vi "VCS Get Motor Parameter.vi"(8 "error in (no error)":errorcluster, 11 "axis in":cluster{"keyHandle":u32, "nodeId":u16}={"keyHandle"=0, "nodeId"=1}) -> (0 "error out":errorcluster, 2 "motor Data":T1={"motor Type"=1, "continuousCurrent"=1000, "peakCurrent"=1000, "polePair"=1, "thermalTimeConstant"=40} {"motor Type" items=["Phase modulated DC motor "=1, "Sinusoidal PM BL motor"=10, "Trapezoidal PM BL motor"=11]}, 3 "axis out":cluster{"keyHandle":u32, "nodeId":u16}={"keyHandle"=0, "nodeId"=1})   [LabVIEW 2017, in "maxonEPOS.lvlib"]
doc: "<B>VCS Get Motor Parameter</B> reads all motor parameters."
uses:
  Examples/maxonEPOS.lvlib
  SSI_Tool/InstrumentsInterfaces/Motordriver/maxon EPOS/Resources/EposCmd.dll
  SSI_Tool/InstrumentsInterfaces/Motordriver/maxon EPOS/Resources/EposCmd64.dll
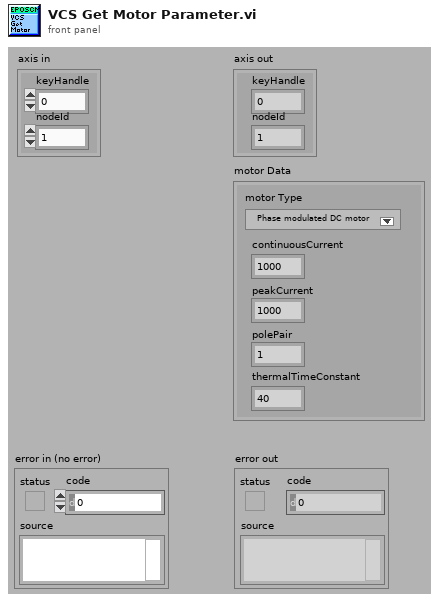
[diagram p1: front panel]
types:
  T1 = cluster{"motor Type":u16, "continuousCurrent":u16, "peakCurrent":u16, "polePair":u8, "thermalTimeConstant":u16}
  T2 = cluster{"pMotorType":u16, "pContinuousCurrent":u16, "pPeakCurrent":u16, "pPolePair":u8, "pThermalTimeConstant":u16}
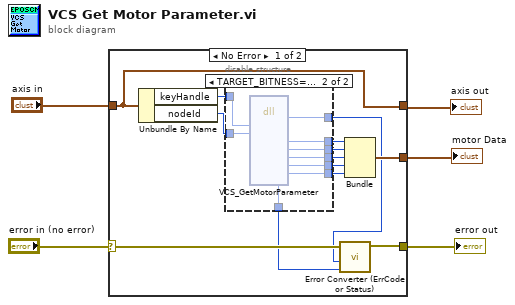
[diagram p0: block diagram]
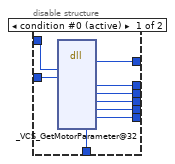
[diagram p2: hidden frame]
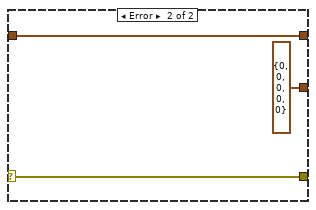
[diagram p3: hidden frame]
diagram:
  n1 = case shown="No Error" "error in (no error)" {
    selector: "error in (no error)" -> [w18 w39]
    tunnel: [w17 w39] -> w4
    tunnel: "axis in" -> [w12 w37]
    tunnel: [w13 T2 {"pMotorType"=0, "pContinuousCurrent"=0, "pPeakCurrent"=0, "pPolePair"=0, "pThermalTimeConstant"=0}] -> w1
    tunnel: [w12 w37] -> w2
    frame No Error {
      n2 = Unbundle By Name(w12) -> ("keyHandle"=w15:u32, "nodeId"=w14:u16)
      n3 = disable-structure shown="TARGET_BITNESS==64" {
        disable-tunnel: [w27 w36] -> w16
        disable-tunnel: w15 -> [w26 w35]
        disable-tunnel: w14 -> [w25 w34]
        disable-tunnel: [w24 w33] -> w11
        disable-tunnel: [w23 w32] -> w10
        disable-tunnel: [w22 w31] -> w9
        disable-tunnel: [w21 w30] -> w8
        disable-tunnel: [w20 w29] -> w7
        disable-tunnel: [w19 w28] -> w6
        frame condition #0 (active) {
          n4 = dll-call lib="C:/workspace/project/scancon/sw/SSI_Tool/InstrumentsInterfaces/Motordriver/maxon EPOS/Resources/EposCmd.*" fn="_VCS_GetMotorParameter@32"("KeyHandle"=w26, "NodeId"=w25) -> (w19:i32, "pMotorType"=w24:u16, "pContinuousCurrent"=w23:u16, "pPeakCurrent"=w22:u16, "pPolePair"=w21:u8, "pThermalTimeConstant"=w20:u16, "pErrorCode"=w27:u32)  [unwired: 11 in, 2 out]
        }
        frame condition #1 {
          n5 = dll-call lib="C:/setup/Resources/EposCmd64.*" fn="VCS_GetMotorParameter" ("EposCmd.dll:_VCS_GetMotorParameter@32")("KeyHandle"=w35, "NodeId"=w34) -> ("Rückgabetyp"=w28:i32, "pMotorType"=w33:u16, "pContinuousCurrent"=w32:u16, "pPeakCurrent"=w31:u16, "pPolePair"=w30:u8, "pThermalTimeConstant"=w29:u16, "pErrorCode"=w36:u32)  [unwired: 11 in, 2 out]
        }
      }
      n6 = call "Error Converter (ErrCode or Status).vi"("error code"=w16, "return type"=w6, "error in (no error)"=w18) -> ("error out"=w17:errorcluster)  [unwired: 7 in]
      n7 = Bundle("pMotorType"=w11, "pContinuousCurrent"=w10, "pPeakCurrent"=w9, "pPolePair"=w8, "pThermalTimeConstant"=w7) -> (w13:T2)  [unwired: 1 in]
    }
    frame Error {
    }
  }
  "error out" <- w4
  "axis out" <- w2
  "motor Data" <- w1
